vi "GE 5565PIORC.VISA.Move In-Place.String (U8).vi"(5 "count (-1: all)":i32=-1, 7 "address space":T1=1 items=["VXI/VME A16"=1, "VXI/VME A24"=2, "VXI/VME A32"=3, "VXI/VME A64"=4, "PXI Memory Allocations"=9, "PXI Configuration"=10, "PXI BAR0"=11, "PXI BAR1"=12, "PXI BAR2"=13, "PXI BAR3"=14, "PXI BAR4"=15, "PXI BAR5"=16], 8 "error in (no error)":errorcluster, 9 "data in":string, 10 "offset":u32, 11 "GE 5565PIORC in":refnum<class "GE 5565PIORC.lvclass">) -> (0 "error out":errorcluster, 1 "data out":string, 3 "GE 5565PIORC out":refnum<class "GE 5565PIORC.lvclass">)   [LabVIEW 2024, in "GE 5565PIORC.lvclass"]
uses:
  GE 5565PIORC.lvclass
  <vilib>/Instr/_visa.llb/VISA Register Access Address Space.ctl
  GE 5565PIORC.lvclass/GE 5565PIORC.ctl
  <vilib>/Utility/error.llb/Error Cluster From Error Code.vi
  visa32.dll
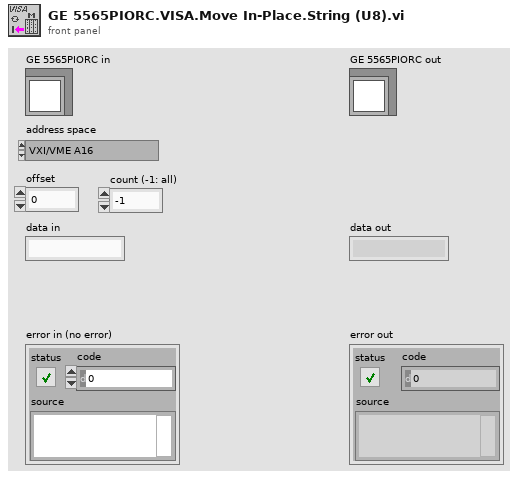
[diagram p1: front panel]
types:
  T1 = typedef "VISA Register Access Address Space.ctl" = u16
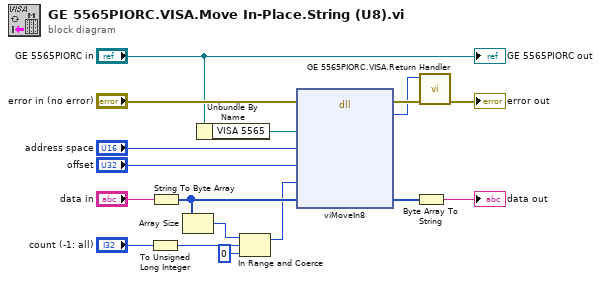
[diagram p0: block diagram]
diagram:
  n1 = To Unsigned Long Integer(number="count (-1: all)") -> (unsigned 32bit integer=w6:u32)
  n2 = String To Byte Array(string="data in") -> (unsigned byte array=w4:u8[])
  n3 = Array Size(array=w4) -> (size(s)=w8:i32)
  n4 = Unbundle By Name("GE 5565PIORC in") -> ("VISA 5565"=w1:refnum<visa-resource-name>)
  n5 = In Range and Coerce(upper limit=w8, x=w6, lower limit=u32 0) -> (coerced(x)=w3:u32)  [unwired: 1 out]
  n6 = dll-call lib="visa32.*" fn="viMoveIn8"(error in="error in (no error)", "session"=w1, "address space"="address space", "offset"="offset", "size"=w3, "data"=w4) -> (error out=w14:errorcluster, "return type"=w12:i32, "data"=w11:u8[])  [unwired: 6 in, 1 out]
  n7 = Byte Array To String(unsigned byte array=w11) -> (string=→"data out":string)
  n8 = call "GE 5565PIORC.VISA.Return Handler.vi"("error in (no error)"=w14, "VISA return value"=w12) -> ("error out"=→"error out":errorcluster)  [unwired: 9 in]
  "GE 5565PIORC out" <- "GE 5565PIORC in"
